vi "Noise (G3)-Initialize.vi"(0 "Noise In":T6, 5 "Level":T4, 7 "Filter":T1={"Type"=enum."Lowpass", "CF (kHz)"=0.0, "BW (kHz)"=0.0, "Cascade"=FALSE, "Quadrature"=FALSE, "Scale Factor"=0.0, "Stages"=[], "Class"=enum."Elliptic", "Order"=0, "BWUnits"=enum."Linear"} {"Stages"."IIR Filter"."Forward Coefficients" format="%.4f"; "Stages"."IIR Filter"."Reverse Coefficients" format="%.4f"}, 9 "Sampling rate (Hz)":dbl, 11 "error in (no error)":errorcluster) -> (4 "Noise Out":T6, 6 "Level Out":T4, 8 "Filter Out":T1={"Type"=enum."Lowpass", "CF (kHz)"=0.0, "BW (kHz)"=0.0, "Cascade"=FALSE, "Quadrature"=FALSE, "Scale Factor"=0.0, "Stages"=[], "Class"=enum."Elliptic", "Order"=0, "BWUnits"=enum."Linear"} {"Stages"."IIR Filter"."Forward Coefficients" format="%.4f"; "Stages"."IIR Filter"."Reverse Coefficients" format="%.4f"}, 10 "Noise":dbl[](array[numeric]), 15 "error out":errorcluster)   [LabVIEW 2020]
uses:
  XControls/Filter (G3)/Filter Data.ctl
  XControls/Filter (G3)/Filter Type.ctl
  Filter VIs/Filter-Bandwidth Units.ctl
  Noise (G3).ctl
  Noise (G3).Properties.ctl
  Noise (G3).Data.ctl
  XControls/Level (G3)/Level Data.ctl
  XControls/Level (G3)/Level Units (G3).ctl
  4th Generation/Classes/Filter/Filter.lvclass/Filter.ctl
  4th Generation/Classes/Filter/Write CF (kHz).vi
  4th Generation/Classes/Filter/Write BW (kHz).vi
  4th Generation/Classes/Filter/Write Units.vi
  4th Generation/Classes/Filter/Write Type.vi
  Waveform VIs/Noise VIs/Noise-Globals.vi
  4th Generation/Classes/Filter/Filter.lvclass
  XControls/Level (G3)/Level (G3).xctl
  XControls/Filter (G3)/Filter (G3).xctl
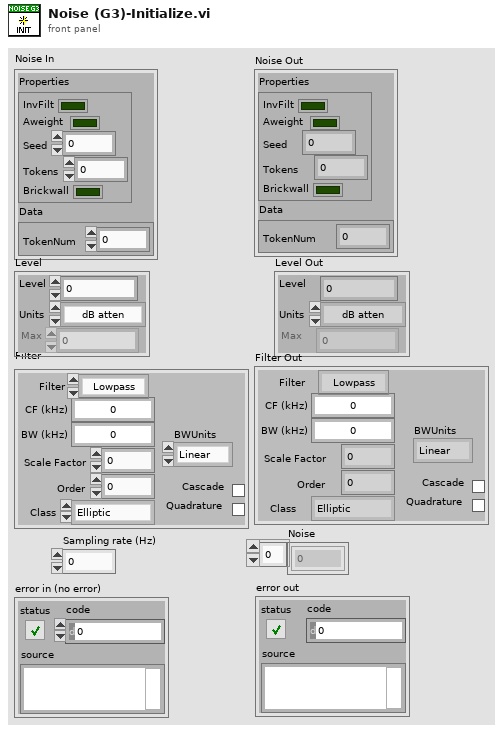
[diagram p1: front panel]
types:
  T1 = typedef "Filter (G3).xctl/Filter Data.ctl" = cluster{"Type":T2, "CF (kHz)":dbl, "BW (kHz)":dbl, "Cascade":bool, "Quadrature":bool, "Scale Factor":dbl, "Stages":cluster{"IIR Filter":cluster{"filter structure":enum32{"IIR 2nd Order", "IIR 4th Order"}, "Reverse Coefficients":dbl[], "Forward Coefficients":dbl[]}, "State":dbl[]}[], "Class":enum16{"Elliptic", "Butterworth"}, "Order":i32, "BWUnits":T3}
  T2 = typedef "Filter (G3).xctl/Filter Type.ctl" = enum16{"OFF", "Lowpass", "Highpass", "Bandpass", "Bandstop"}
  T3 = typedef "Filter-Bandwidth Units.ctl" = enum16{"Linear", "Octaves", "Min-Max"}
  T4 = typedef "Level (G3).xctl/Level Data.ctl" = cluster{"Level":dbl, "Units":T5, "Max":dbl, "Data":cluster{"Multiplier":dbl, "Cal File":path, "Cal":cluster{"Freq (Hz)":dbl[], "Mag (dB SPL)":dbl[], "Phase (deg)":dbl[]}, "audiogram":path}}
  T5 = typedef "Level (G3).xctl/Level Units (G3).ctl" = enum16{"dB atten", "dB SPL", "dB re 1 Vrms", "dB V/Hz½", "mW", "dB HL", "Volts", "dB mW"}
  T6 = typedef "Noise (G3).ctl" = cluster{"Properties":T7, "Data":T8}
  T7 = typedef "Noise (G3).Properties.ctl" = cluster{"InvFilt":bool, "Aweight":bool, "Seed":i32, "Tokens":i32, "Brickwall":bool}
  T8 = typedef "Noise (G3).Data.ctl" = cluster{"TokenNum":i32}
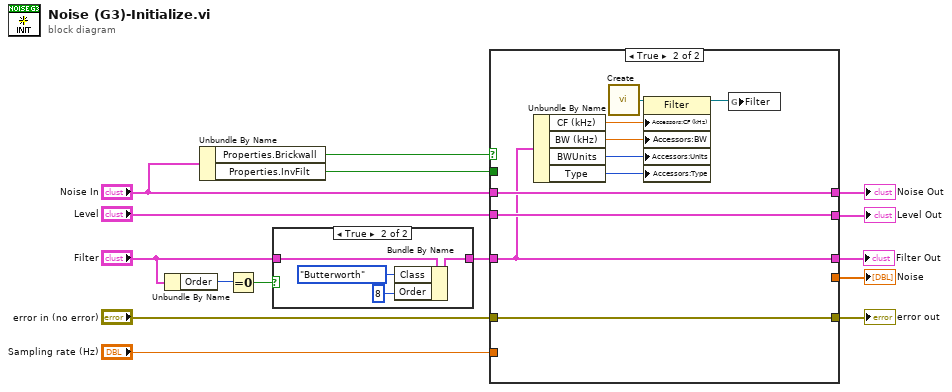
[diagram p0: block diagram]
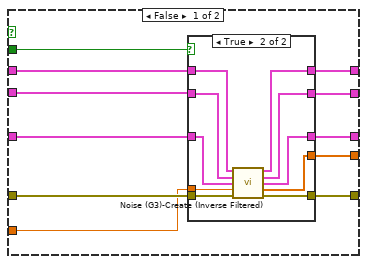
[diagram p2: hidden frame]
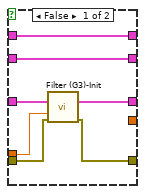
[diagram p3: hidden frame]
diagram:
  n1 = Unbundle By Name("Filter") -> ("Order"=w5:i32)
  n2 = Unbundle By Name("Noise In") -> ("Properties.Brickwall"=w1:bool, "Properties.InvFilt"=w8:bool)
  n3 = Equal To 0?(x=w5) -> (x = 0?=w3:bool)
  n4 = case shown="True" w3 {
    tunnel: "Filter" -> [w16 w20]
    tunnel: [w16 w19] -> w2
    frame False {
    }
    frame True {
      n5 = Bundle By Name(cluster=w20, "Class"=enum16{"Elliptic", "Butterworth"}."Butterworth", "Order"=8) -> (w19:T1)
    }
  }
  n6 = case shown="True" w1 {
    tunnel: "error in (no error)" -> [w31 w57]
    tunnel: [w30 w57] -> w14
    tunnel: "Sampling rate (Hz)" -> [w29 _]
    tunnel: [w28 w55] -> w12
    tunnel: [w27 _] -> w11
    tunnel: [w26 w56] -> w10
    tunnel: [w25 w58] -> w9
    tunnel: w8 -> [w24 _]
    tunnel: "Level" -> [w23 w58]
    tunnel: "Noise In" -> [w22 w56]
    tunnel: w2 -> [w21 w55]
    frame False {
      n7 = case shown="True" w24 {
        tunnel: w29 -> [w38 w46]
        tunnel: w31 -> [w37 w48]
        tunnel: [w34 w45] -> w26
        tunnel: [w36 w47] -> w30
        tunnel: w22 -> [w34 w40]
        tunnel: w23 -> [w33 w41]
        tunnel: [w33 w44] -> w25
        tunnel: [w35 w43] -> w28
        tunnel: [_ w42] -> w27
        tunnel: w21 -> [w32 w39]
        frame False {
          n8 = call "Filter (G3)-Init.vi"("Filter"=w32, "Sampling rate (Hz)"=w38, "error in (no error)"=w37) -> ("Filter out"=w35:T1, "error out"=w36:errorcluster)  [unwired: 11 in]
        }
        frame True {
          n9 = call "Noise (G3)-Create (Inverse Filtered).vi"("Noise In"=w40, "Level In"=w41, "Filter In"=w39, "Fs (Hz)"=w46, "error in (no error)"=w48) -> ("Noise Out"=w45:T6, "Level Out"=w44:T4, "Filter Out"=w43:T1, "InvFilter Noise"=w42:dbl[], "error out"=w47:errorcluster)  [unwired: 6 in]
        }
      }
    }
    frame True {
      n10 = Unbundle By Name(w55) -> ("CF (kHz)"=w53:dbl, "BW (kHz)"=w52:dbl, "BWUnits"=w51:T3, "Type"=w50:T2)
      n11 = call "Create.vi"() -> ("Filter"=w54:refnum<class "Filter.lvclass">)  [unwired: 15 in]
      n12 = property class="Filter"(reference=w54, "Accessors:CF (kHz)"=w53, "Accessors:BW"=w52, "Accessors:Units"=w51, "Accessors:Type"=w50) -> (reference out=w49:refnum<class "Filter.lvclass">)  [unwired: 1 in, 1 out]
      n13 = global write "Noise-Globals.vi" "Filter"(w49) -> ()
    }
  }
  "error out" <- w14
  "Noise Out" <- w10
  "Level Out" <- w9
  "Filter Out" <- w12
  "Noise" <- w11
